vi "Notify Match Failed.vi"(8 "error in":errorcluster, 10 "SDO abort code":T1 items=["Toggle bit not allowed"=84082688, "SDO protocol timed out"=84148224, "Client/server command specifier not valid or unknown"=84148225, "Invalid block size (block mode only)"=84148226, "Invalid sequence number (block mode only)"=84148227, "CRC error (block mode only)"=84148228, "Out of memory"=84148229, "Attempt to read a write only object"=100728833, "Attempt to write a read only object"=100728834, "Object does not exist in the object dictionary"=100794368, "Object cannot be mapped to the PDO"=100925505, "The number and length of the objects to be mapped would exceed PDO length"=100925506, "General parameter incompatibility reason"=100925507, "General internal incompatibility in the device"=100925511, "Access failed due to an hardware error"=101056512, "Data type does not match, length of service parameter does not match"=101122064, "Data type does not match, length of service parameter too high"=101122066, "Data type does not match, length of service parameter too low"=101122067, "Sub-index does not exist"=101253137, "Invalid value for parameter (download only)"=101253168, "Value of parameter written too high (download only)"=101253169, "Value of parameter written too low (download only)"=101253170, "Maximum value is less than minimum value"=101253174, "Resource not available: SDO connection"=101318691, "General error"=134217728, "Data cannot be transferred or stored to the application"=134217760, "Data cannot be transferred or stored to the application because of local control"=134217761, "Data cannot be transferred or stored to the application because of the present device stable"=134217762, "Object dictionary dynamic generation fails or no object dictionary is present (e.g. object dictionary is generated from file and generation fails because of an file error)"=134217763, "No data available"=134217764], 11 "SDO Transfer in":refnum<class "SDO Transfer.lvclass">) -> (0 "error out":errorcluster, 3 "SDO Transfer out":refnum<class "SDO Transfer.lvclass">)   [LabVIEW 2020, in "CANopen.lvlib" / "SDO Manager.lvlib" / "SDO Transfer.lvclass"]
uses:
  SDO Transfer.lvclass
  SDO Transfer.lvclass/SDO Transfer.ctl
  SDO abort code.ctl
  Typedefs/SDO Result.ctl
  SDO Transfer Result.ctl
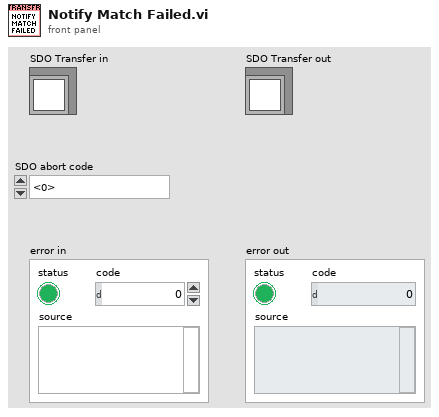
[diagram p1: front panel]
types:
  T1 = typedef "CANopen.lvlib/SDO Manager.lvlib/SDO Transfer.lvclass/SDO abort code.ctl" = u32
  T2 = typedef "CANopen.lvlib/SDO Manager.lvlib/SDO Transfer.lvclass/SDO Transfer Result.ctl" = cluster{"SDO Result":T3, "Error":errorcluster}
  T3 = typedef "CANopen.lvlib/SDO Manager.lvlib/SDO Transfer.lvclass/SDO Result.ctl" = cluster{"Success":bool, "SDO abort code":cluster{"Null":bool, "Value":T1}, "Data":cluster{"Null":bool, "Data":u8[]}}
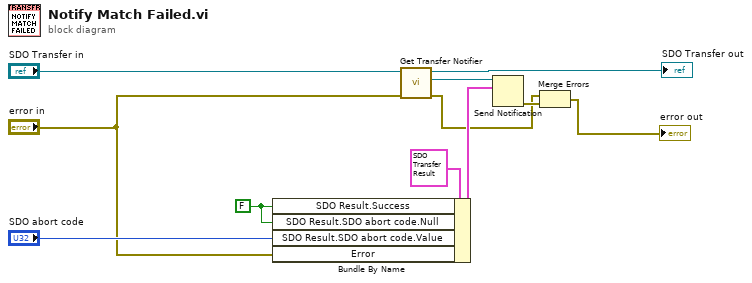
[diagram p0: block diagram]
diagram:
  w10 = FALSE ("SDO Result.Success")
  n1 = Bundle By Name(cluster=T2 {"SDO Result"={"Success"=FALSE, "SDO abort code"={"Null"=TRUE, "Value"=84082688}, "Data"={"Null"=TRUE, "Data"=[]}}, "Error"={"status"=FALSE, "code"=0, "source"=""}} ("notification"), "SDO Result.Success"=w10, "SDO Result.SDO abort code.Null"=w10, "SDO Result.SDO abort code.Value"="SDO abort code", "Error"="error in") -> (w7:T2)
  n2 = call "Get Transfer Notifier.vi"("error in"="error in", "SDO Transfer in"="SDO Transfer in") -> ("error out"=w2:errorcluster, "SDO Transfer Notifier"=w3:refnum<notifier>, "SDO Transfer out"=→"SDO Transfer out":refnum<class "SDO Transfer.lvclass">)  [unwired: 7 in]
  n3 = Send Notification(notification=w7, notifier=w3) -> (error out=w4:errorcluster)  [unwired: 1 in, 1 out]
  n4 = Merge Errors(w2, w4) -> (→"error out":errorcluster)
